vi "StateMachine2.vi"() -> ()   [LabVIEW 2014]
uses:
  testMachineCtr.ctl
  testStateMachineCtr.ctl
panel:
  in  "stop":bool
  out "data":dbl format="%#.6g"
  in  "exitButton":bool
  out "stateTest":T1
  out "ensaio":bool
  in  "waiting time":u32
  in  "currentCycleCtr":u32
  out "freio":bool
  in  "velocidade 2":u32
  out "velocidade":u32
  out "motor":bool
  in  "velocidade_inferior":u32
  in  "velocidade_superior":u32
  out "totalCycle":string
  out "currentCycle":string
  in  "numberOfCycles":u32 max=999 step=1 format="%0d"
  in  "stopButton":bool
  in  "startButton":bool
  out "state":T2
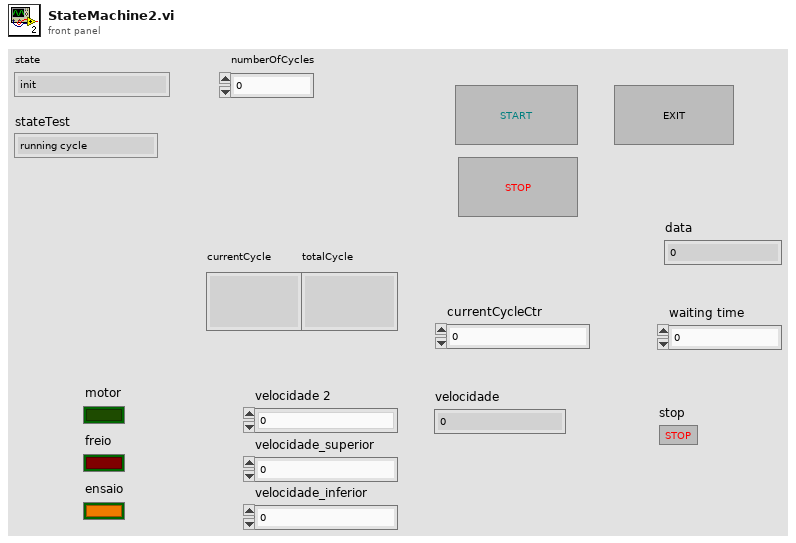
[diagram p1: front panel]
types:
  T1 = typedef "testStateMachineCtr.ctl" = enum16{"running cycle", "acquiring data", "braking cycle", "stopping cycle"}
  T2 = typedef "testMachineCtr.ctl" = enum16{"init", "ready", "running", "stopped", "finish", "shutdown"}
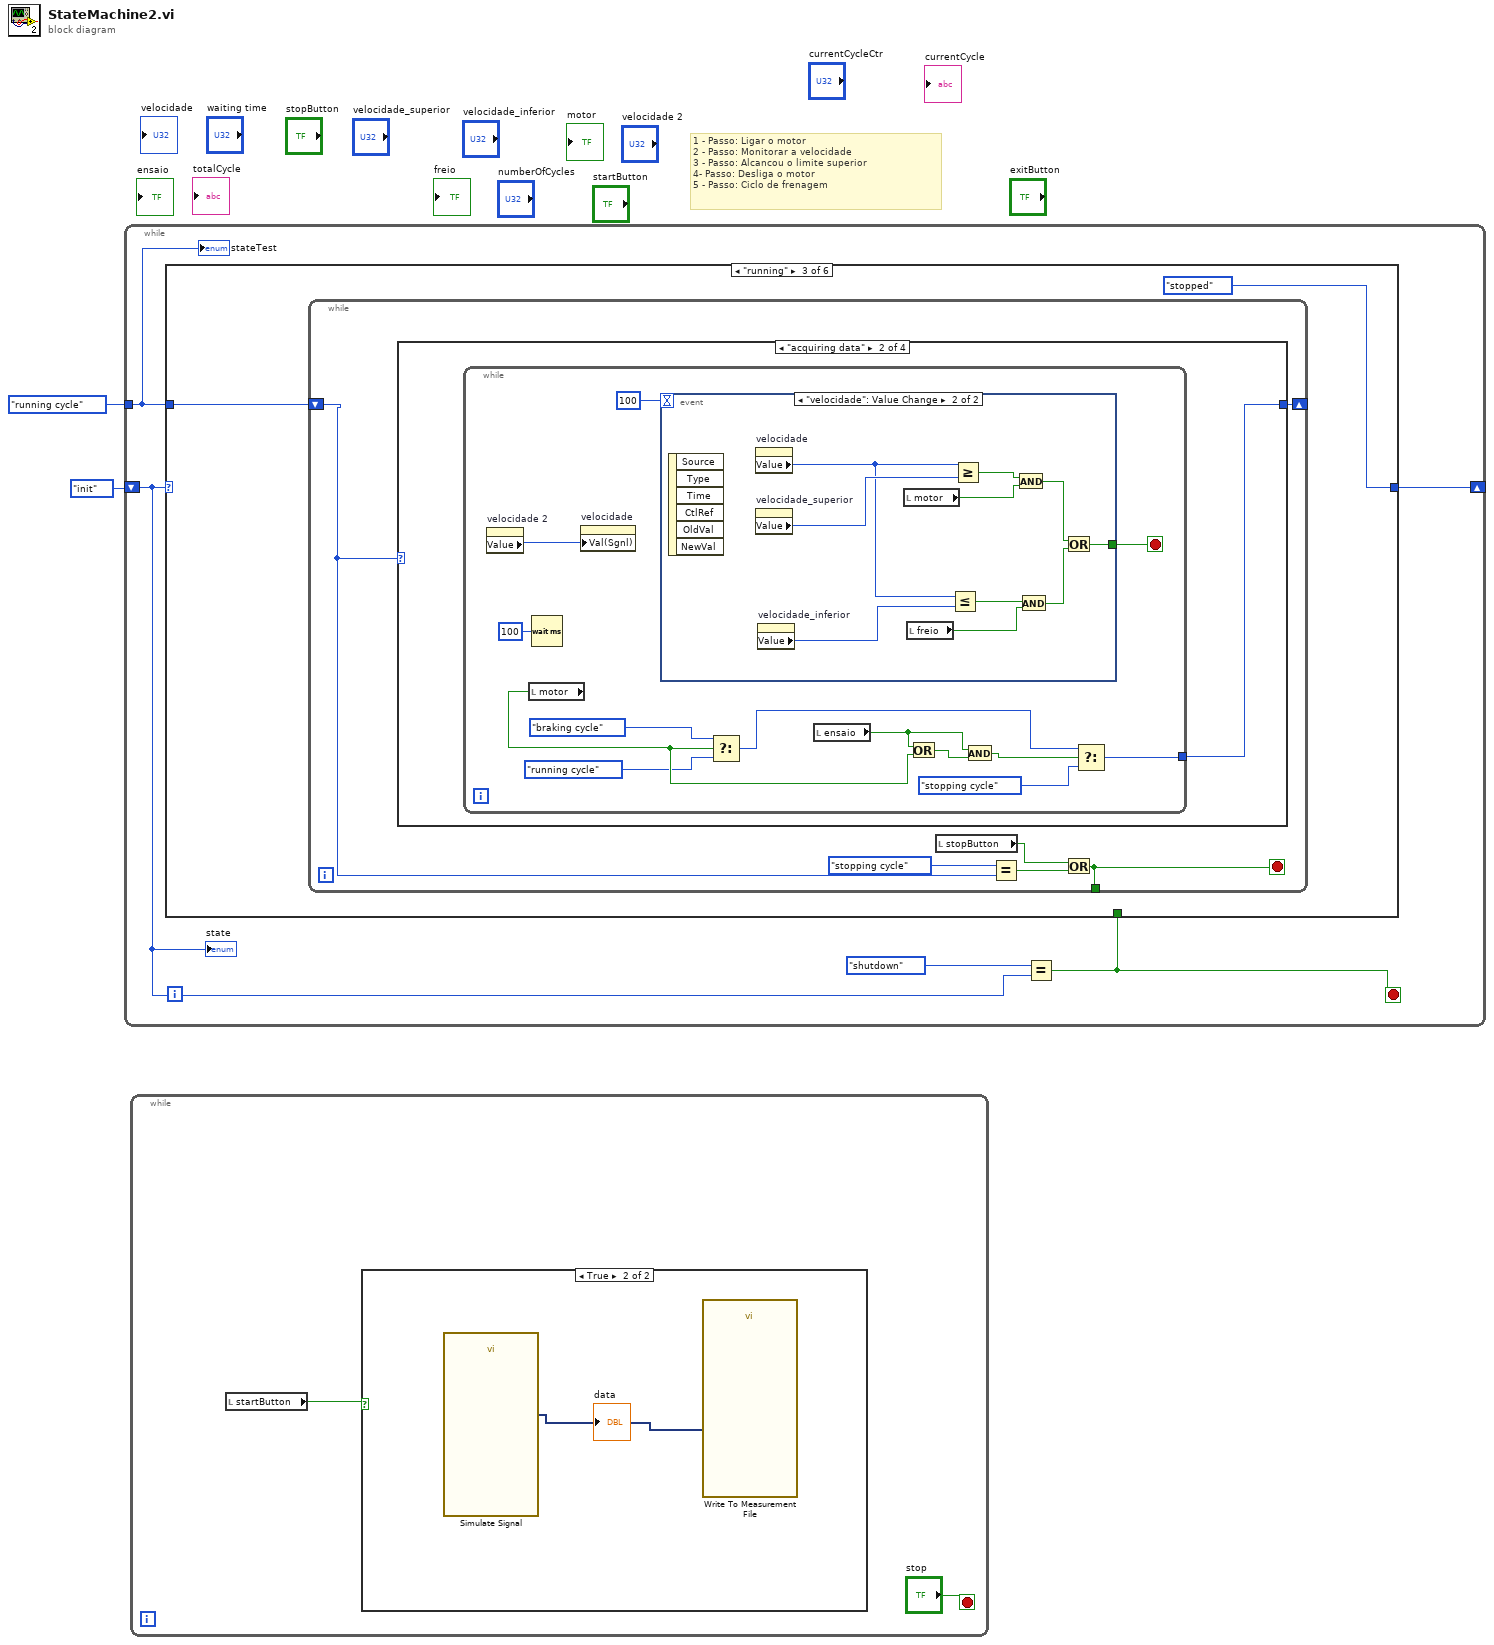
[diagram p0: block diagram]
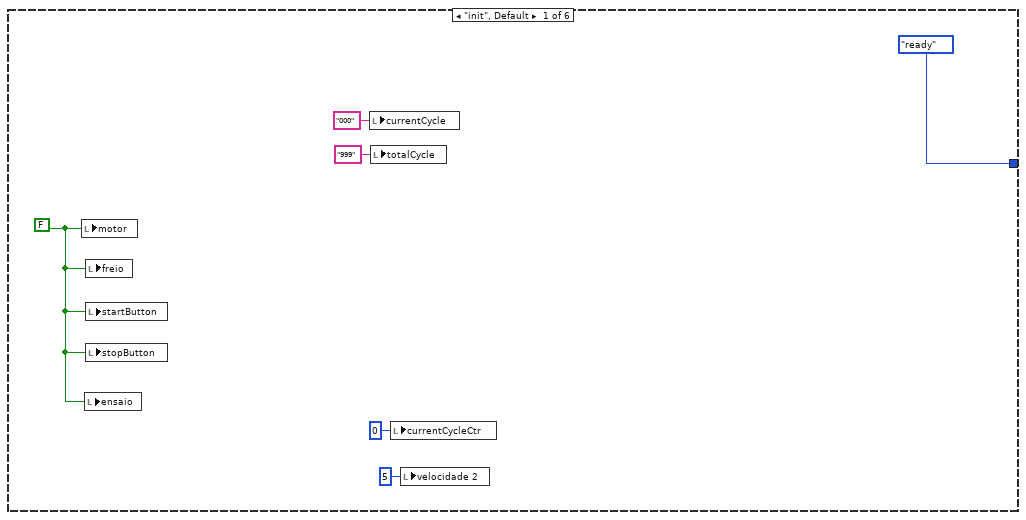
[diagram p3: hidden frame]
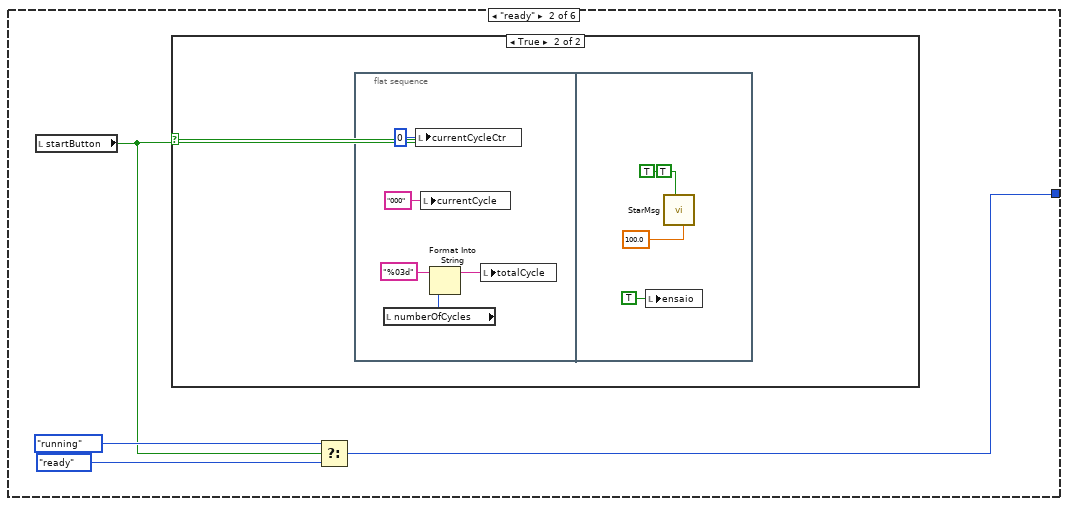
[diagram p4: hidden frame]
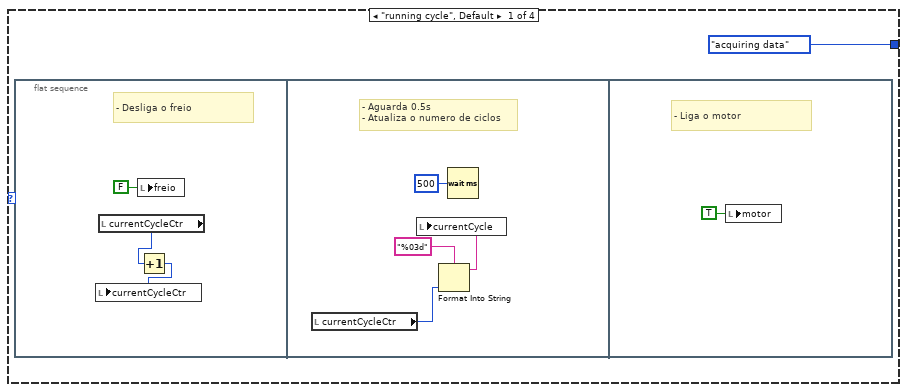
[diagram p6: hidden frame]
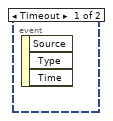
[diagram p7: hidden frame]
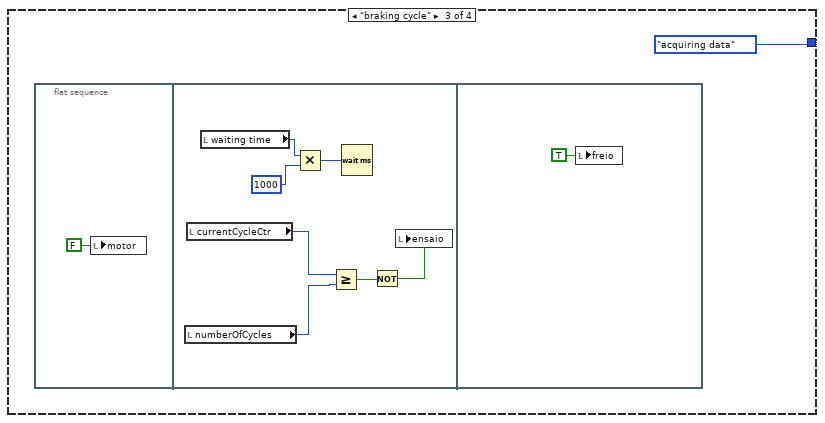
[diagram p8: hidden frame]
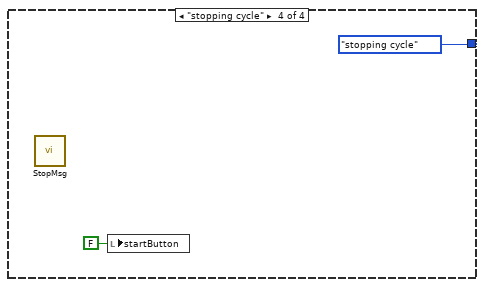
[diagram p9: hidden frame]
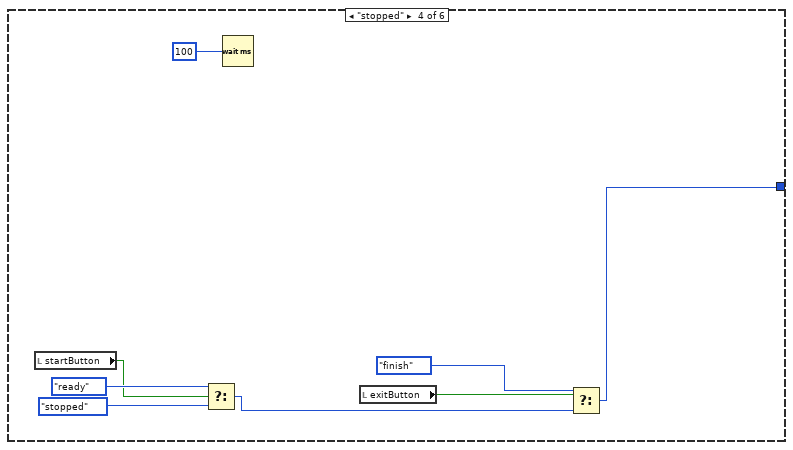
[diagram p10: hidden frame]
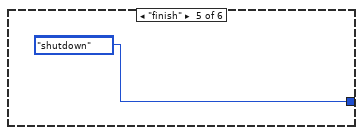
[diagram p11: hidden frame]
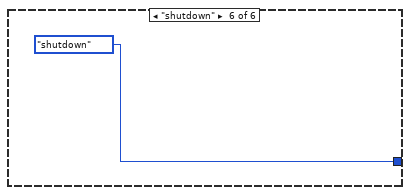
[diagram p12: hidden frame]
diagram:
  # "1 - Passo: Ligar o motor\n2 - Passo: Monitorar a velocidade\n3 - Passo: Alcancou o limite superior\n4- Passo: Desliga o motor\n5 - Passo: Ciclo de frenagem"
  n1 = while {
    shift-right: [w5] -> _
    shift-left: testMachineCtr."init" ("state") -> [w7]
    tunnel: testStateMachineCtr."running cycle" ("stateTest") -> [w4]
    stop <- w3 stop-if-true
    n2 = Equal?(x=testMachineCtr."shutdown" ("state"), y=w7) -> (x = y?=w3:bool)
    n3 = case shown="\"running\"" w7 {
      tunnel: w3 -> [_ _ _ _ _ _]
      tunnel: [testMachineCtr."ready" ("state") w15 testMachineCtr."stopped" ("state") w83 testMachineCtr."shutdown" ("state") testMachineCtr."shutdown" ("state")] -> w5
      tunnel: w4 -> [_ _ w26 _ _ _]
      frame "init", Default {
        w11 = FALSE ("motor")
        n4 = local write "motor"(w11) -> ()
        n5 = local write "ensaio"(w11) -> ()
        n6 = local write "freio"(w11) -> ()
        n7 = local write "startButton"(w11) -> ()
        n8 = local write "stopButton"(w11) -> ()
        n9 = local write "currentCycle"("000" ("currentCycle")) -> ()
        n10 = local write "totalCycle"("999" ("totalCycle")) -> ()
        n11 = local write "currentCycleCtr"(u32 0 ("currentCycleCtr")) -> ()
        n12 = local write "velocidade 2"(u32 5 ("velocidade 2")) -> ()
      }
      frame "ready" {
        n13 = local read "startButton"() -> (w14:bool)
        n14 = case shown="True" w14 {
          frame False {
          }
          frame True {
            n15 = flat-sequence {
              frame #0 {
                n16 = local read "numberOfCycles"() -> (w20:u32)
                n17 = local write "currentCycleCtr"(u32 0 ("currentCycleCtr")) -> ()
                n18 = local write "currentCycle"("000" ("currentCycle")) -> ()
                n19 = Format Into String(format string="%03d", w20) -> (resulting string=w21:string)  [unwired: 2 in, 1 out]
                n20 = local write "totalCycle"(w21) -> ()
              }
              frame #1 {
                (unwired) TRUE ("Cancel Button (True)")
                n21 = local write "ensaio"(TRUE ("ensaio")) -> ()
                n22 = call "StarMsg.vi"("Show"=TRUE, "Max Value (100)"=100.0) -> ()  [unwired: 7 in, 2 out]
              }
            }
          }
        }
        n23 = Select(t=testMachineCtr."running" ("state"), s=w14, f=testMachineCtr."ready" ("state")) -> (s? t:f=w15:T2)
      }
      frame "running" {
        n24 = while {
          shift-right: [w32] -> _
          shift-left: w26 -> [w29]
          tunnel: [w28] -> _
          stop <- w28 stop-if-true
          n25 = case shown="\"acquiring data\"" w29 {
            tunnel: [testStateMachineCtr."acquiring data" ("stateTest") w43 testStateMachineCtr."acquiring data" ("stateTest") testStateMachineCtr."stopping cycle" ("stateTest")] -> w32
            frame "running cycle", Default {
              n26 = flat-sequence {
                frame #0 {
                  # "- Desliga o freio"
                  n27 = local read "currentCycleCtr"() -> (w36:u32)
                  n28 = local write "freio"(FALSE ("freio")) -> ()
                  n29 = Increment(x=w36) -> (x+1=w35:u32)
                  n30 = local write "currentCycleCtr"(w35) -> ()
                }
                frame #1 {
                  # "- Aguarda 0.5s \n- Atualiza o numero de ciclos"
                  n31 = local read "currentCycleCtr"() -> (w38:u32)
                  n32 = Format Into String(format string="%03d", w38) -> (resulting string=w39:string)  [unwired: 2 in, 1 out]
                  n33 = local write "currentCycle"(w39) -> ()
                  n34 = Wait (ms)(milliseconds to wait=u32 500) -> ()  [unwired: 1 out]
                }
                frame #2 {
                  # "- Liga o motor"
                  n35 = local write "motor"(TRUE ("motor")) -> ()
                }
              }
            }
            frame "acquiring data" {
              n36 = while {
                tunnel: [w47] -> w43
                stop <- w53 stop-if-true
                n37 = property on="velocidade 2" class="DigNum (strict)"() -> ("Value"=w54:u32)  [unwired: 2 in, 2 out]
                n38 = local read "motor"() -> (w51:bool)
                n39 = Wait (ms)(milliseconds to wait=u32 100) -> ()  [unwired: 1 out]
                n40 = property on="velocidade" class="DigNum (strict)"("Val(Sgnl)"=w54) -> ()  [unwired: 2 in, 2 out]
                n41 = event shown="[1] \"velocidade\": Value Change" {
                  selector: _ -> [_ _]
                  dyn-events: _ -> [_ _]
                  timeout: 100 -> [_ _]
                  tunnel: [_ w57] -> w53
                  event Timeout {
                    n42 = event-data() -> ()  [unwired: 1 in, 3 out]
                  }
                  event "velocidade": Value Change {
                    n43 = event-data() -> ()  [unwired: 1 in, 6 out]
                    n44 = property on="velocidade" class="DigNum (strict)"() -> ("Value"=w63:u32)  [unwired: 2 in, 2 out]
                    n45 = property on="velocidade_superior" class="DigNum (strict)"() -> ("Value"=w66:u32)  [unwired: 2 in, 2 out]
                    n46 = property on="velocidade_inferior" class="DigNum (strict)"() -> ("Value"=w62:u32)  [unwired: 2 in, 2 out]
                    n47 = local read "motor"() -> (w64:bool)
                    n48 = local read "freio"() -> (w61:bool)
                    n49 = Less Or Equal?(x=w63, y=w62) -> (x <= y?=w60:bool)
                    n50 = Greater Or Equal?(x=w63, y=w66) -> (x >= y?=w65:bool)
                    n51 = And(x=w65, y=w64) -> (x .and. y?=w58:bool)
                    n52 = And(x=w60, y=w61) -> (x .and. y?=w59:bool)
                    n53 = Or(x=w58, y=w59) -> (x .or. y?=w57:bool)
                  }
                }
                n54 = Select(t=testStateMachineCtr."braking cycle" ("stateTest"), s=w51, f=testStateMachineCtr."running cycle" ("stateTest")) -> (s? t:f=w52:T1)
                n55 = local read "ensaio"() -> (w50:bool)
                n56 = Or(x=w50, y=w51) -> (x .or. y?=w49:bool)
                n57 = And(x=w50, y=w49) -> (x .and. y?=w48:bool)
                n58 = Select(t=w52, s=w48, f=testStateMachineCtr."stopping cycle" ("stateTest")) -> (s? t:f=w47:T1)
              }
            }
            frame "braking cycle" {
              n59 = flat-sequence {
                frame #0 {
                  n60 = local write "motor"(FALSE ("motor")) -> ()
                }
                frame #1 {
                  n61 = local read "numberOfCycles"() -> (w71:u32)
                  n62 = local read "currentCycleCtr"() -> (w72:u32)
                  n63 = local read "waiting time"() -> (w75:u32)
                  n64 = Multiply(x=w75, y=u32 1000) -> (x*y=w73:u32)
                  n65 = Greater Or Equal?(x=w72, y=w71) -> (x >= y?=w70:bool)
                  n66 = Wait (ms)(milliseconds to wait=w73) -> ()  [unwired: 1 out]
                  n67 = Not(x=w70) -> (.not. x?=w69:bool)
                  n68 = local write "ensaio"(w69) -> ()
                }
                frame #2 {
                  n69 = local write "freio"(TRUE ("freio")) -> ()
                }
              }
            }
            frame "stopping cycle" {
              n70 = call "StopMsg.vi"() -> ()  [unwired: 9 in, 2 out]
              n71 = local write "startButton"(FALSE ("startButton")) -> ()
            }
          }
          n72 = local read "stopButton"() -> (w30:bool)
          n73 = Equal?(x=testStateMachineCtr."stopping cycle" ("stateTest"), y=w29) -> (x = y?=w31:bool)
          n74 = Or(x=w30, y=w31) -> (x .or. y?=w28:bool)
        }
      }
      frame "stopped" {
        n75 = local read "startButton"() -> (w84:bool)
        n76 = Select(t=testMachineCtr."ready" ("state"), s=w84, f=testMachineCtr."stopped" ("state")) -> (s? t:f=w80:T2)
        n77 = Wait (ms)(milliseconds to wait=u32 100) -> ()  [unwired: 1 out]
        n78 = local read "exitButton"() -> (w79:bool)
        n79 = Select(t=testMachineCtr."finish" ("state"), s=w79, f=w80) -> (s? t:f=w83:T2)
      }
      frame "finish" {
        (unwired) testMachineCtr."shutdown" ("state")
      }
      frame "shutdown" {
      }
    }
    "state" <- w7
    "stateTest" <- w4
  }
  n80 = while {
    stop <- "stop" stop-if-true
    n81 = local read "startButton"() -> (w89:bool)
    n82 = case shown="True" w89 {
      frame False {
      }
      frame True {
        n83 = call "Simulate Signal"() -> ("Sine"=w91:dynamicdata)  [unwired: 14 in, 1 out]
        "data" <- w91
        n84 = call "Write To Measurement File"("Signals"=w91) -> ()  [unwired: 16 in, 3 out]
      }
    }
  }
